vi "System Version.vi"(8 "error in (no error)":errorcluster, 11 "VISA resource name":refnum<visa-resource-name>) -> (0 "error out":errorcluster, 2 "System Version":string, 3 "VISA resource name out":refnum<visa-resource-name>)   [LabVIEW 2020, in "Rohde&Schwarz CMXP GPRF.lvlib"]
doc: "This VI queries the number of the SCPI version, which is relevant for the instrument.\n\nAttribute:\nRSCMXPGPRF_ATTR_SYSTEM_VERSION\n\nRemote-control command:\nSYSTem:VERSion?"
uses:
  <instrlib>/Rohde&Schwarz CMXP GPRF/Rohde&Schwarz CMXP GPRF.lvlib
  Instance           1 32Saved   rscmwgprf System Version .vi
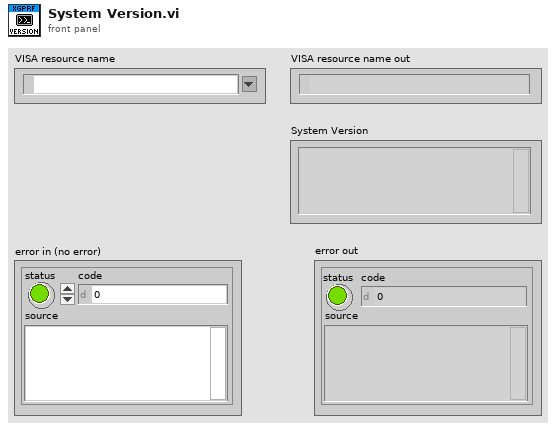
[diagram p1: front panel]
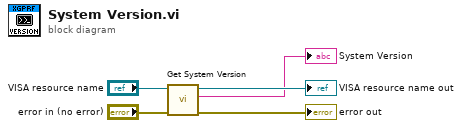
[diagram p0: block diagram]
diagram:
  n1 = call "Get System Version"("error in (no error)"="error in (no error)", "instrument handle"="VISA resource name") -> ("error out"=→"error out":errorcluster, "System Version"=→"System Version":string, "instrument handle out"=→"VISA resource name out":refnum<visa-resource-name>)  [unwired: 7 in]
